vi "GEOM_FindReadMode.vi"(8 "error in (no error)":errorcluster, 10 "Detector":T7 {"ReadModes"."amplifiers"."fliped" items=["none", "horizontal", "vertical"]; "ReadModes"."amplifiers"."type" items=["LL", "LR", "UL", "UR"]}, 11 "ReadMode name":string) -> (0 "error out":errorcluster, 1 "empty":bool, 2 "ReadMode":T2 {"amplifiers"."fliped" items=["none", "horizontal", "vertical"]; "amplifiers"."type" items=["LL", "LR", "UL", "UR"]}, 3 "found?":bool, 4 "detector":T1)   [LabVIEW 2016]
uses:
  GEOM_DetStruct.ctl
  GEOM_ReadMode.ctl
  GEOM_Amplifier.ctl
  GEOM_AmpType.ctl
  GEOM_ROI.ctl
  GEOM_Coords.ctl
  GEOM_DetSummaryStruct.ctl
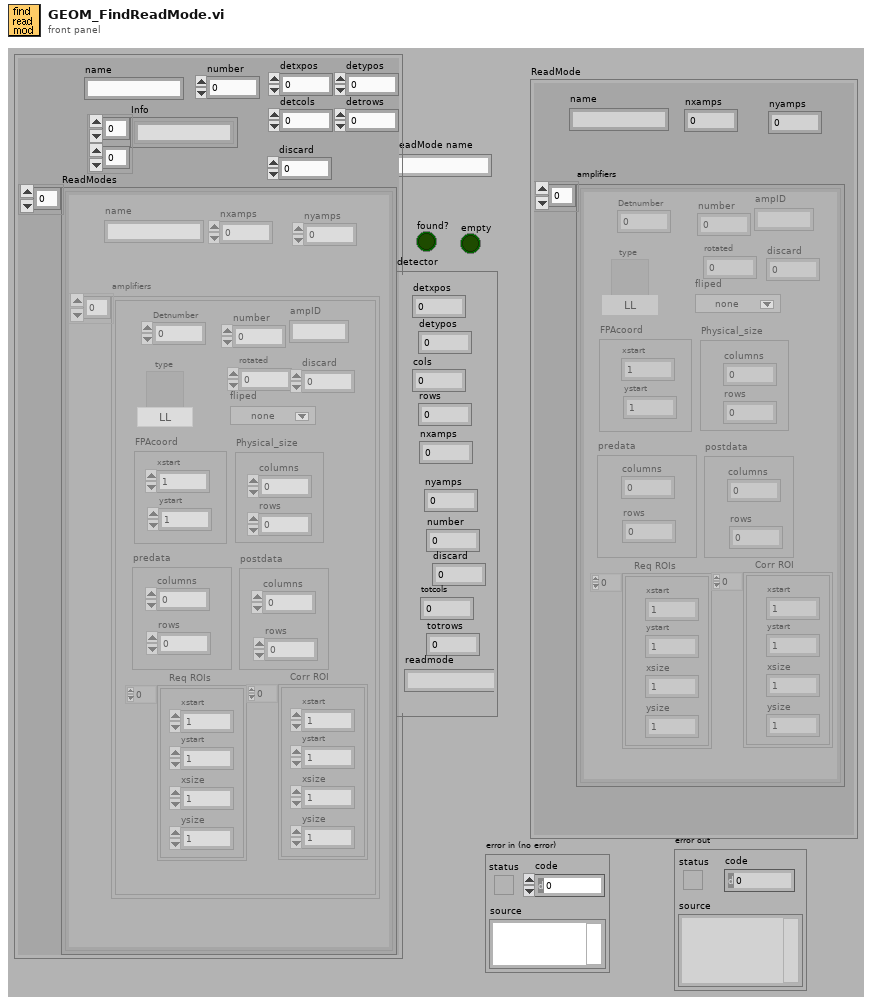
[diagram p1: front panel]
types:
  T1 = typedef "GEOM_DetSummaryStruct.ctl" = cluster{"detxpos":i32, "detypos":i32, "cols":i32, "rows":i32, "nxamps":i32, "nyamps":i32, "number":i32, "discard":i32, "totcols":i32, "totrows":i32, "readmode":string}
  T2 = typedef "GEOM_ReadMode.ctl" = cluster{"name":string, "amplifiers":T3[], "nxamps":i32, "nyamps":i32}
  T3 = typedef "GEOM_Amplifier.ctl" = cluster{"number":i32, "type":T4, "rotated":i16, "fliped":u16, "FPAcoord":cluster{"xstart":i32, "ystart":i32}, "Physical_size":cluster{"columns":i32, "rows":i32}, "predata":cluster{"columns":i32, "rows":i32}, "postdata":cluster{"columns":i32, "rows":i32}, "Req ROIs":T5, "Corr ROI":T5, "Detnumber":i32, "ampID":string, "discard":i32}
  T4 = typedef "GEOM_AmpType.ctl" = u16
  T5 = typedef "GEOM_ROI.ctl" = T6[]
  T6 = typedef "GEOM_Coords.ctl" = cluster{"xstart":u32, "ystart":u32, "xsize":u32, "ysize":u32}
  T7 = typedef "GEOM_DetStruct.ctl" = cluster{"name":string, "number":i32, "Info":string[][], "ReadModes":T2[], "detxpos":i32, "detypos":i32, "detcols":i32, "detrows":i32, "discard":i32}
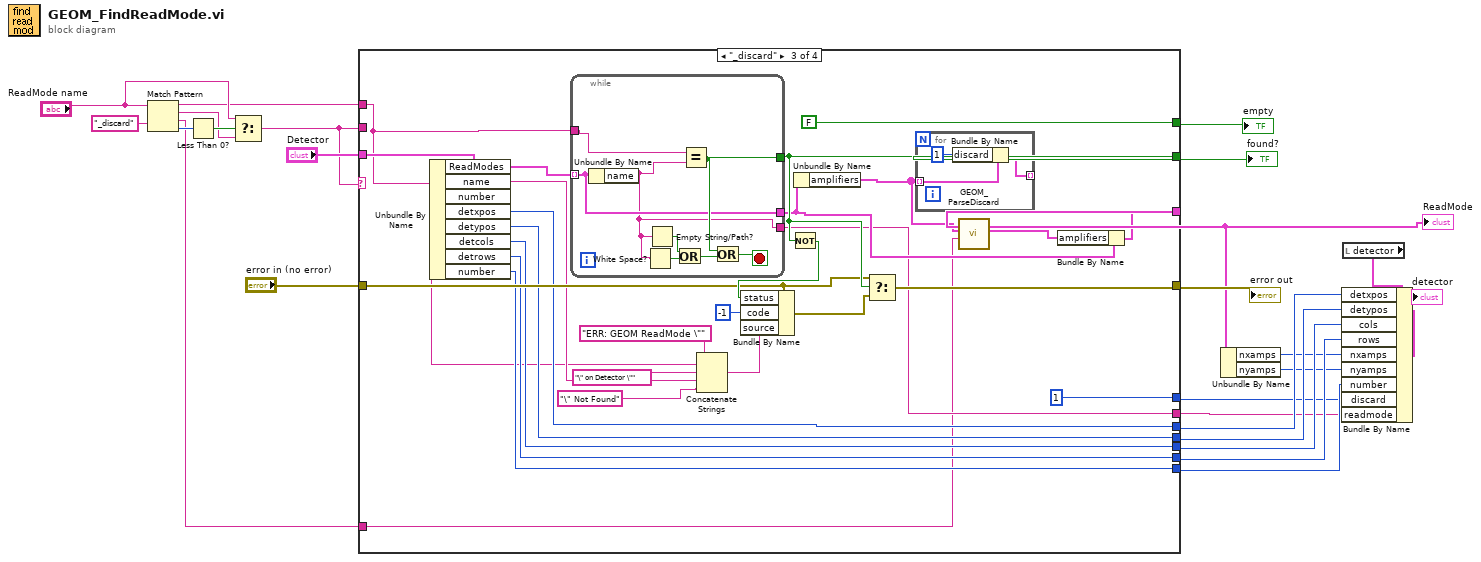
[diagram p0: block diagram]
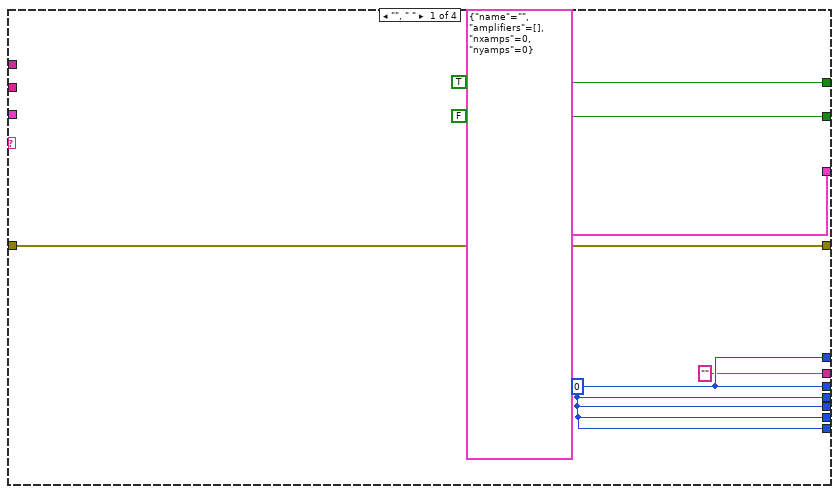
[diagram p2: hidden frame]
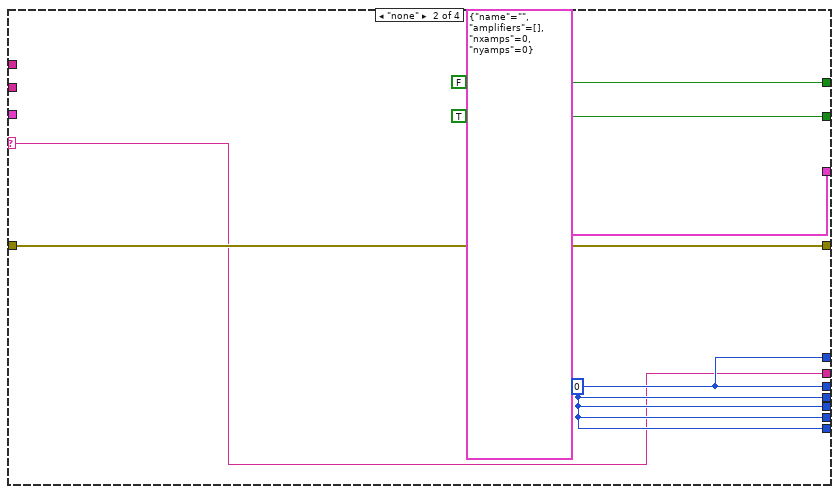
[diagram p3: hidden frame]
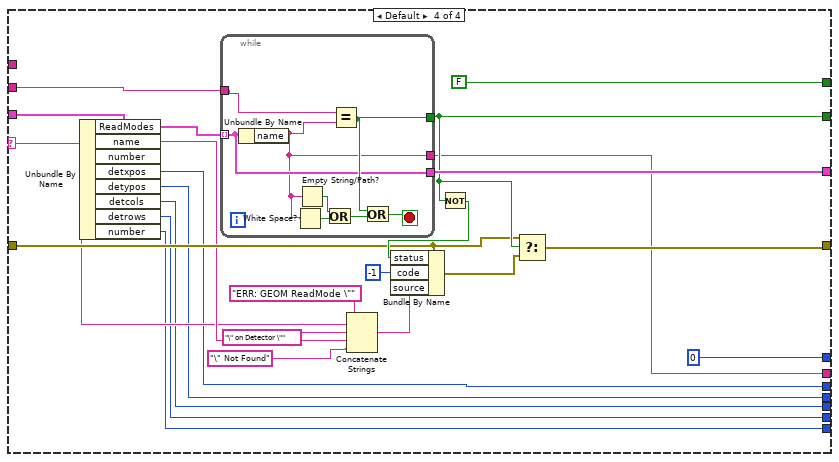
[diagram p4: hidden frame]
diagram:
  n1 = Match Pattern(string="ReadMode name", regular expression="_discard") -> (before substring=w4:string, match substring=w5:string, after substring=w1:string, offset past match=w9:i32)  [unwired: 1 out]
  n2 = Less Than 0?(x=w9) -> (x < 0?=w8:bool)
  n3 = Select(t="ReadMode name", s=w8, f=w5) -> (s? t:f=w6:string)
  n4 = case shown="\"_discard\"" w6 {
    selector: w6 -> [_ w32 _ w84]
    tunnel: w6 -> [_ _ _ w99]
    tunnel: [FALSE TRUE w59 w92] -> w25
    tunnel: [T2 {"name"="", "amplifiers"=[], "nxamps"=0, "nyamps"=0} ("ReadMode") T2 {"name"="", "amplifiers"=[], "nxamps"=0, "nyamps"=0} ("ReadMode") w43 w97] -> w16
    tunnel: [TRUE FALSE FALSE FALSE] -> w24
    tunnel: "error in (no error)" -> [w29 w35 w58 w91]
    tunnel: [w29 w35 w56 w89] -> w22
    tunnel: [w27 w33 w51 w83] -> w20
    tunnel: [w27 w33 w50 w82] -> w19
    tunnel: [w27 w33 w49 w81] -> w18
    tunnel: [w27 w33 w48 w80] -> w17
    tunnel: [w27 w33 w46 w79] -> w12
    tunnel: "Detector" -> [_ _ w47 w78]
    tunnel: w4 -> [_ _ w42 _]
    tunnel: [w27 w33 1 ("discard") 0 ("discard")] -> w3
    tunnel: ["" ("name") w32 w41 w76] -> w2
    tunnel: w1 -> [_ _ w39 _]
    frame "", " " {
      w27 = 0 ("detxpos")
    }
    frame "none" {
      w33 = 0 ("detxpos")
    }
    frame "_discard" {
      n5 = Unbundle By Name(w47) -> ("ReadModes"=w64:T2[], "name"=w53:string, "detxpos"=w51:i32, "detypos"=w50:i32, "detcols"=w49:i32, "detrows"=w48:i32, "number"=w46:i32)  [unwired: 1 out]
      n6 = while {
        tunnel: w42 -> [w75]
        tunnel: w64 -> [w73] mode=indexing
        tunnel: [w74] -> w59
        tunnel: [w73] -> w44
        tunnel: [w68] -> w41
        stop <- w69 stop-if-true
        n7 = Unbundle By Name(w73) -> ("name"=w68:string)
        n8 = White Space?(1:w68) -> (0:w71:bool)
        n9 = Empty String/Path?(string/path=w68) -> (empty?=w72:bool)
        n10 = Or(x=w72, y=w71) -> (x .or. y?=w70:bool)
        n11 = Equal?(x=w75, y=w68) -> (x = y?=w74:bool)
        n12 = Or(x=w74, y=w70) -> (x .or. y?=w69:bool)
      }
      n13 = Concatenate Strings("ERR: GEOM ReadMode \"", w42, "\" on Detector \"", w53, "\" Not Found") -> (w60:string)
      n14 = Not(x=w59) -> (.not. x?=w62:bool)
      n15 = Bundle By Name(cluster=w58, "status"=w62, "code"=-1, "source"=w60) -> (w57:errorcluster)
      n16 = Unbundle By Name(w44) -> ("amplifiers"=w40:T3[])
      n17 = Select(t=w58, s=w59, f=w57) -> (s? t:f=w56:errorcluster)
      n18 = for {
        tunnel: w40 -> [w67] mode=indexing
        tunnel: [w65] -> _ mode=indexing
        n19 = Bundle By Name(cluster=w67, "discard"=1) -> (w65:T3)
      }
      n20 = call "GEOM_ParseDiscard.vi"("discard args"=w39, "amplifiers"=w40) -> ("amplifiers out"=w38:T3[])  [unwired: 9 out]
      n21 = Bundle By Name(cluster=w44, "amplifiers"=w38) -> (w43:T2)
    }
    frame Default {
      n22 = Unbundle By Name(w78) -> ("ReadModes"=w98:T2[], "name"=w86:string, "detxpos"=w83:i32, "detypos"=w82:i32, "detcols"=w81:i32, "detrows"=w80:i32, "number"=w79:i32)  [unwired: 1 out]
      n23 = while {
        tunnel: w99 -> [w107]
        tunnel: w98 -> [w105] mode=indexing
        tunnel: [w106] -> w92
        tunnel: [w105] -> w97
        tunnel: [w100] -> w76
        stop <- w101 stop-if-true
        n24 = Unbundle By Name(w105) -> ("name"=w100:string)
        n25 = White Space?(1:w100) -> (0:w103:bool)
        n26 = Empty String/Path?(string/path=w100) -> (empty?=w104:bool)
        n27 = Or(x=w104, y=w103) -> (x .or. y?=w102:bool)
        n28 = Equal?(x=w107, y=w100) -> (x = y?=w106:bool)
        n29 = Or(x=w106, y=w102) -> (x .or. y?=w101:bool)
      }
      n30 = Concatenate Strings("ERR: GEOM ReadMode \"", w84, "\" on Detector \"", w86, "\" Not Found") -> (w93:string)
      n31 = Not(x=w92) -> (.not. x?=w95:bool)
      n32 = Bundle By Name(cluster=w91, "status"=w95, "code"=-1, "source"=w93) -> (w90:errorcluster)
      n33 = Select(t=w91, s=w92, f=w90) -> (s? t:f=w89:errorcluster)
    }
  }
  "found?" <- w25
  "ReadMode" <- w16
  "empty" <- w24
  "error out" <- w22
  n34 = Unbundle By Name(w16) -> ("nxamps"=w15:i32, "nyamps"=w14:i32)
  n35 = local read "detector"() -> (w21:T1)
  n36 = Bundle By Name(cluster=w21, "detxpos"=w20, "detypos"=w19, "cols"=w18, "rows"=w17, "nxamps"=w15, "nyamps"=w14, "number"=w12, "discard"=w3, "readmode"=w2) -> (→"detector":T1)
